vi "ep_Convert Spectra.vi"(8 "error in (no error)":errorcluster, 9 "fundamental frequency [Hz]":dbl=50.0, 10 "slip":dbl, 11 "spectra":T3) -> (0 "error out":errorcluster, 2 "search information":T1, 3 "spectra points":T2)   [LabVIEW 2014, in "NI_EP_Motor Monitoring.lvlib"]
uses:
  <vilib>/addons/Electrical Power/Motor Monitoring/NI_EP_Motor Monitoring.lvlib
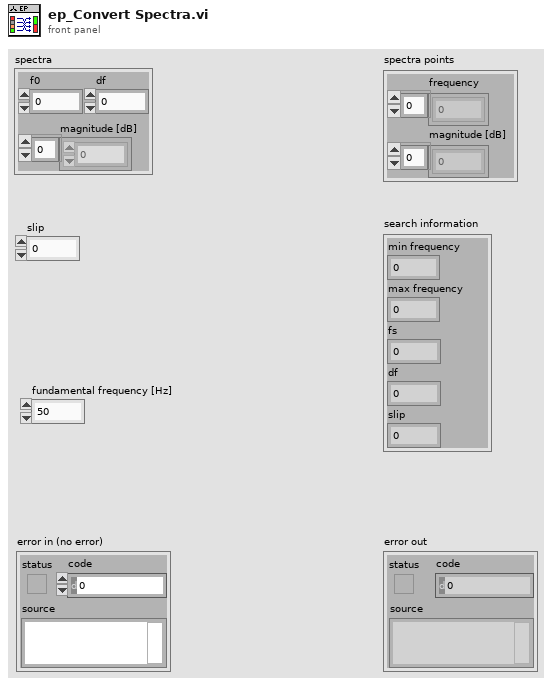
[diagram p1: front panel]
types:
  T1 = cluster{"min frequency":dbl, "max frequency":dbl, "fs":dbl, "df":dbl, "slip":dbl}
  T2 = cluster{"frequency":dbl[], "magnitude [dB]":dbl[]}
  T3 = cluster{"f0":dbl, "df":dbl, "magnitude [dB]":dbl[]}
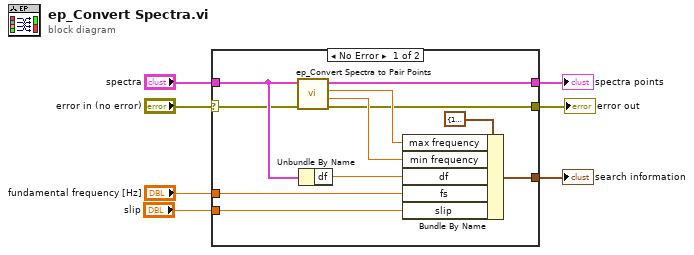
[diagram p0: block diagram]
diagram:
  n1 = case shown="No Error" "error in (no error)" {
    selector: "error in (no error)" -> [w10 w19]
    tunnel: "spectra" -> [w12 _]
    tunnel: [w18 _] -> w6
    tunnel: [w9 w19] -> w2
    tunnel: "slip" -> [w8 _]
    tunnel: "fundamental frequency [Hz]" -> [w16 _]
    tunnel: [w15 _] -> w3
    frame No Error {
      n2 = call <vilib>:"ep_Convert Spectra to Pair Points.vi"("error in (no error)"=w10, "spectra"=w12) -> ("error out"=w9:errorcluster, "min frequency"=w13:dbl, "max frequency"=w14:dbl, "spectra points"=w18:T2)  [unwired: 6 in]
      n3 = Unbundle By Name(w12) -> ("df"=w11:dbl)
      n4 = Bundle By Name(cluster=T1 {"min frequency"=1.0, "max frequency"=1.0, "fs"=0.0, "df"=0.02, "slip"=0.0} ("relevant parameters"), "max frequency"=w14, "min frequency"=w13, "df"=w11, "fs"=w16, "slip"=w8) -> (w15:T1)
    }
    frame Error {
    }
  }
  "spectra points" <- w6
  "search information" <- w3
  "error out" <- w2
